vi "Average_P_step.vi"(6 "Averaged P(B) in":dbl[][](array[numeric]), 7 "B array":dbl[](array[numeric]), 9 "Up/Down":bool, 10 "Counter":i8, 11 "Stepped P(B)":dbl[][](array[numeric])) -> (3 "Averaged P(B) out":dbl[][](array[numeric]))   [LabVIEW 2015]
panel:
  out "element":dbl
  out "Offset array dn":dbl[](array[numeric])
  out "P(B) Stepped 2":cluster{"B array":dbl[], "Stepped P(B)":dbl[]}[](graph)
  out "P(B) Averaged":cluster{"B array":dbl[], dbl[]}[](graph)
  out "P(B) Offset removed":cluster{"B array":dbl[], "Stepped P(B)":dbl[]}[](graph)
  out "P(B) Stepped":cluster{"B array":dbl[], dbl[]}[](graph)
  out "OffsetRemoved":dbl[][](array[numeric])
  out "Offset array":dbl[](array[numeric])
  out "size(s)":i32
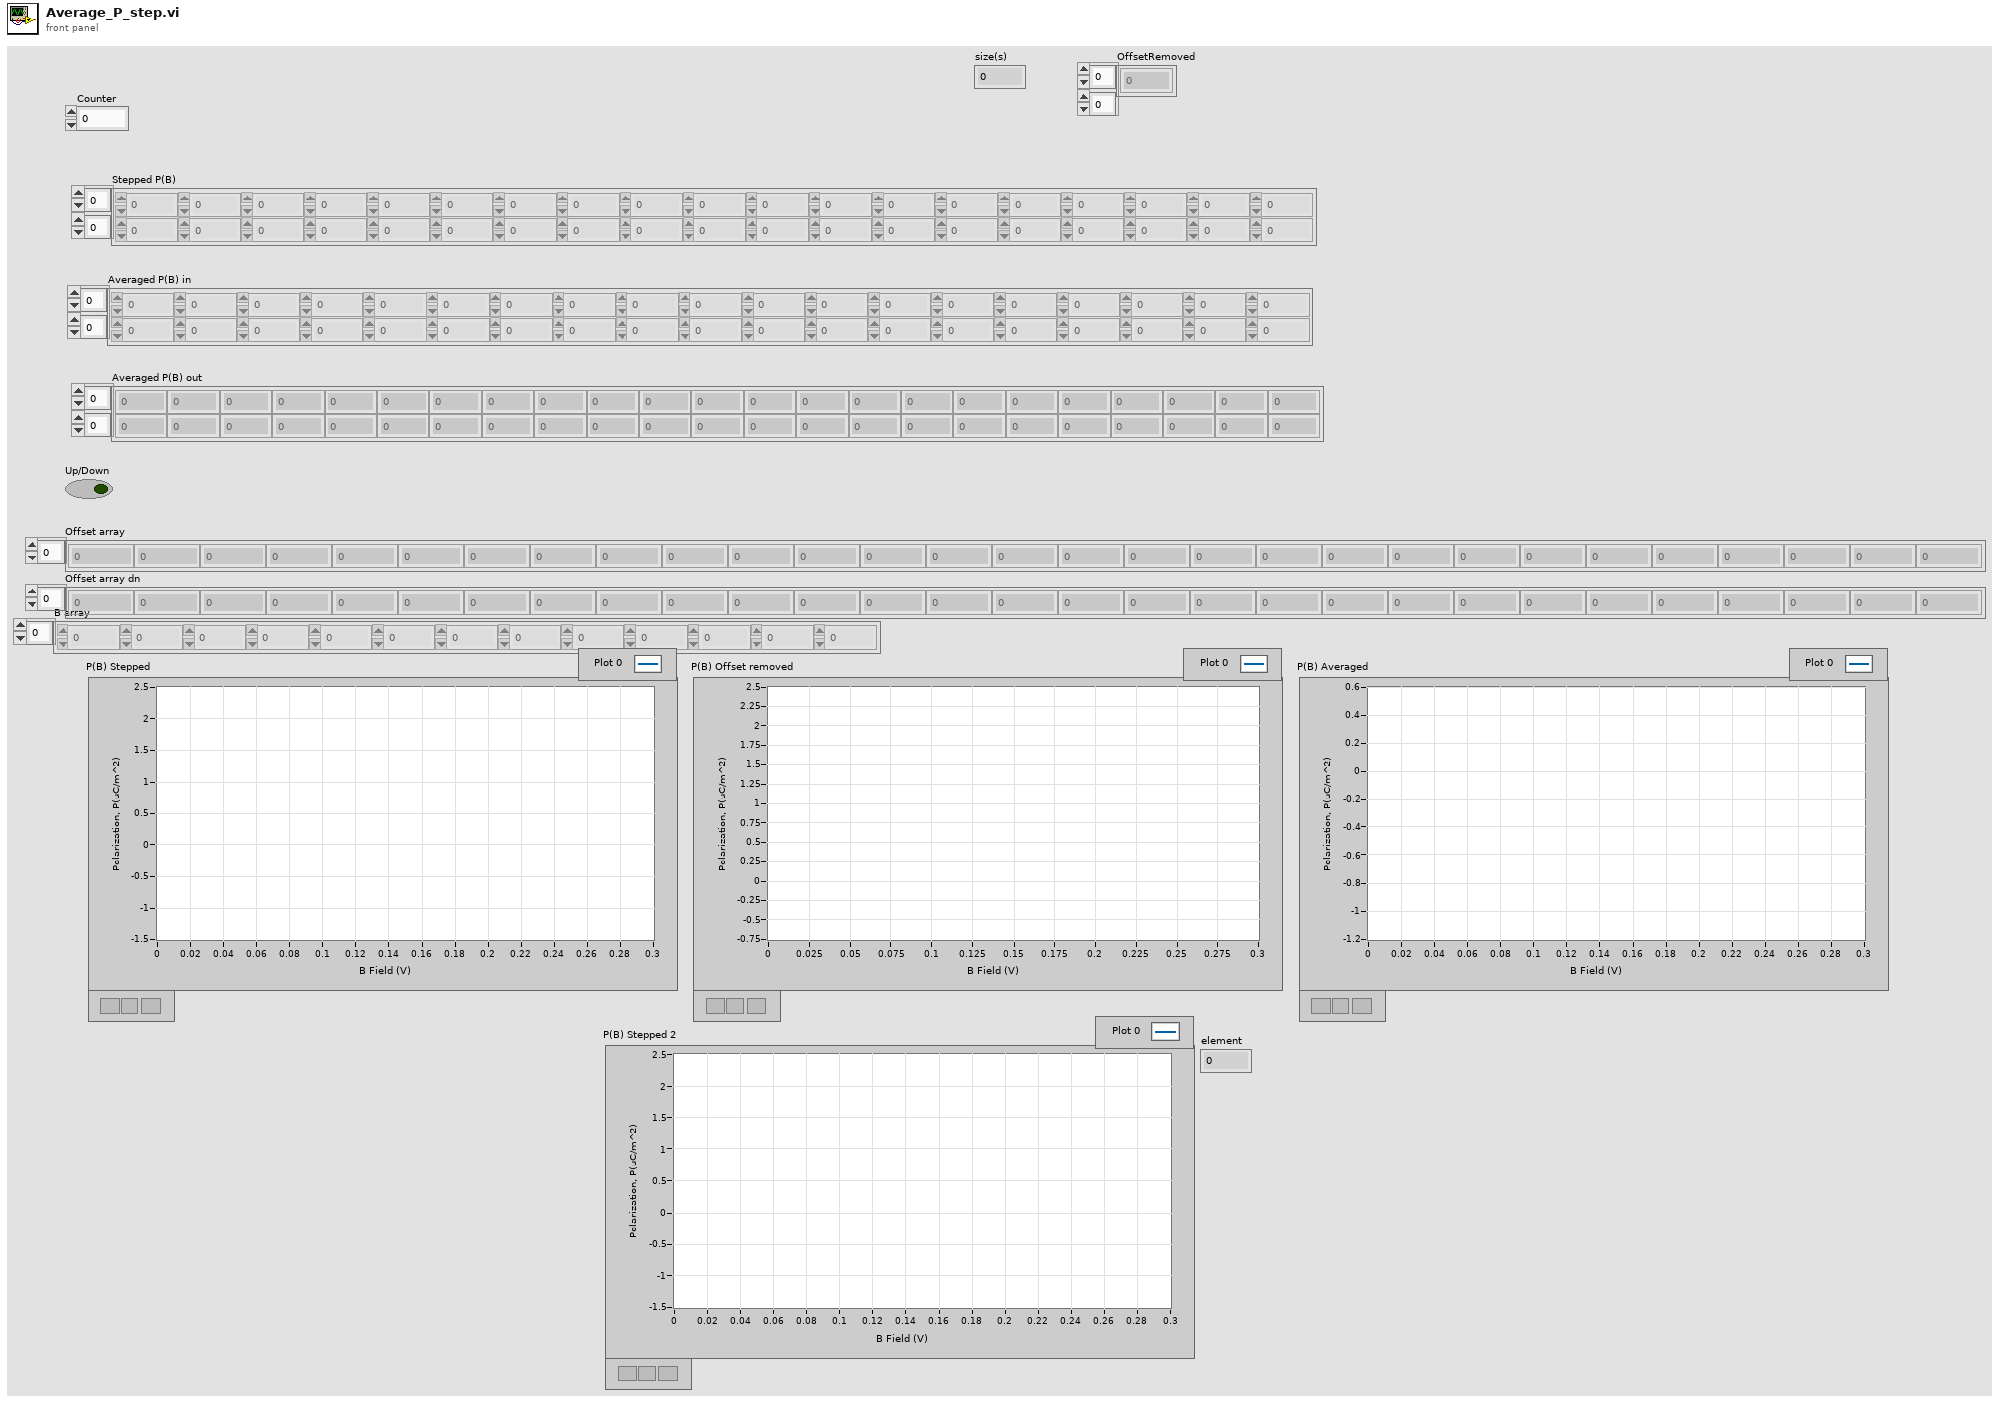
[diagram p1: front panel]
types:
  T1 = cluster{"B array":dbl[], "Averaged P(B) in":dbl[]}
  T2 = cluster{"B array":dbl[], "Averaged P(B) in":dbl[]}[]
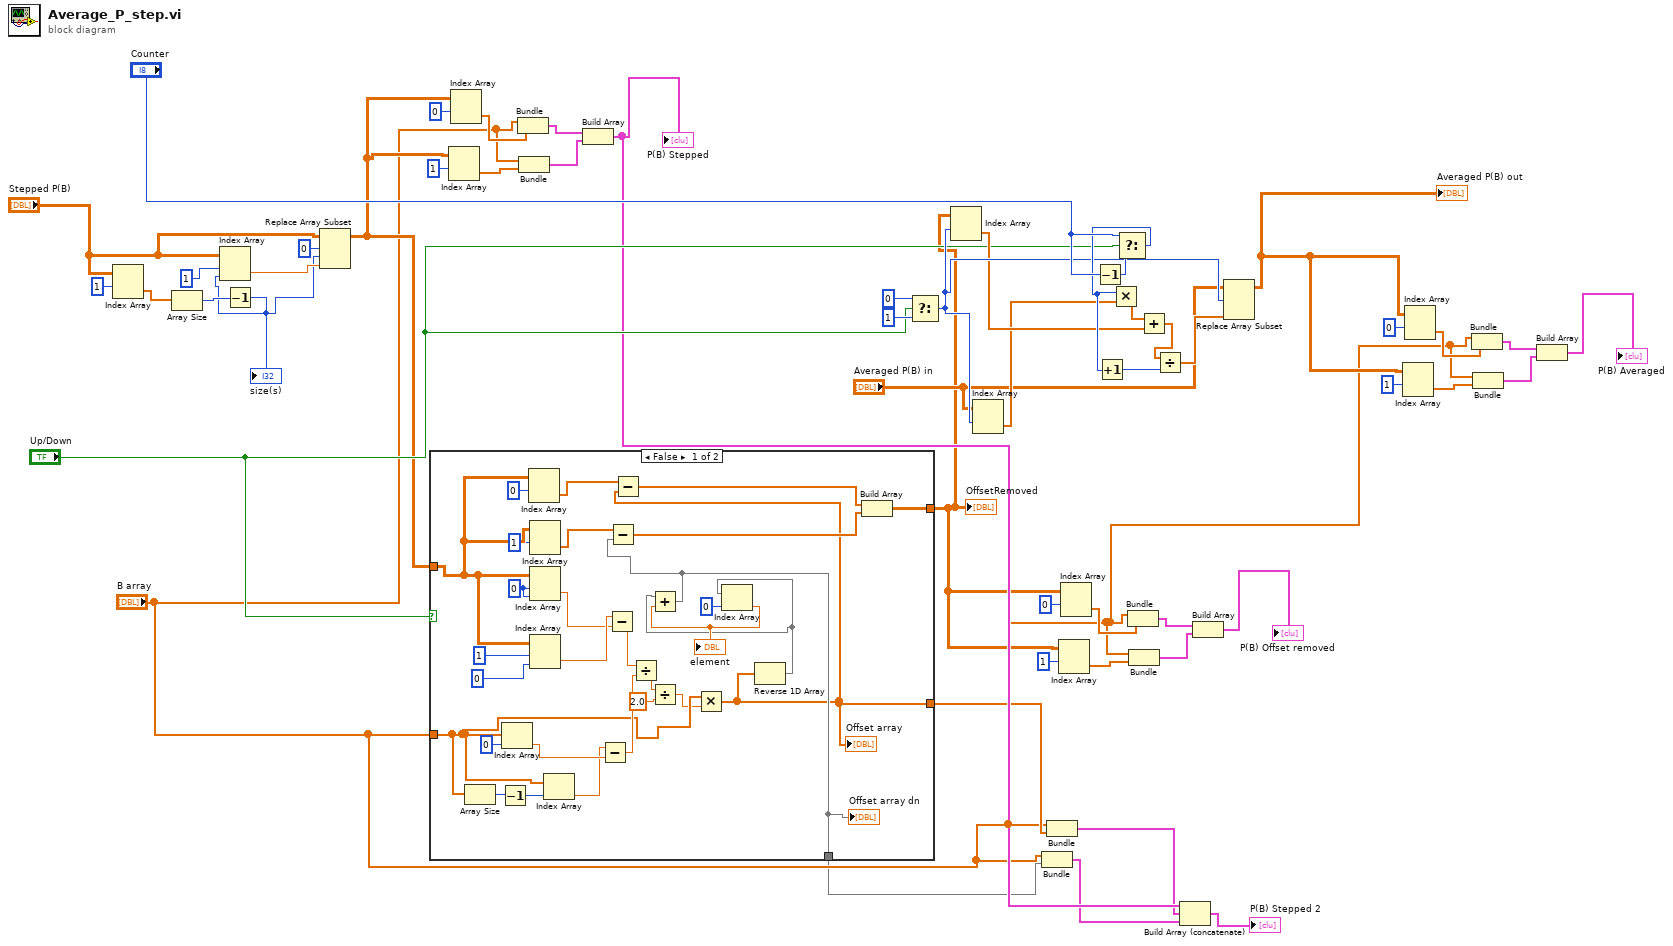
[diagram p0: block diagram]
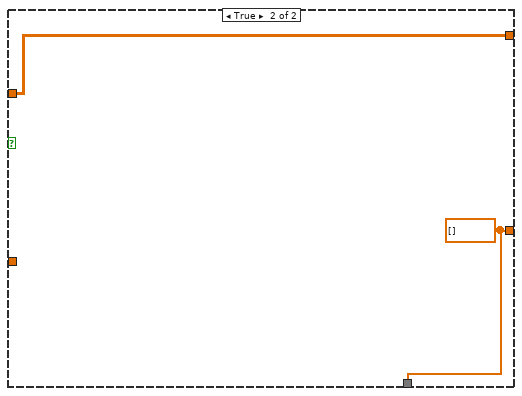
[diagram p2: hidden frame]
diagram:
  n1 = Index Array(array="Stepped P(B)", index (row)=1) -> (element=w39:dbl[])  [unwired: 1 in]
  n2 = Array Size(array=w39) -> (size(s)=w36:i32)
  n3 = Decrement(x=w36) -> (x-1=w33:i32)
  "size(s)" <- w33
  n4 = Index Array(array="Stepped P(B)", index (row)=1, index (col)=w33) -> (element=w37:dbl)
  n5 = Replace Array Subset(array="Stepped P(B)", new element=w37, index (row)=0, index (col)=w33) -> (w9:dbl[][])
  n6 = case shown="False" "Up/Down" {
    tunnel: w9 -> [w73 w83]
    tunnel: "B array" -> [w60 _]
    tunnel: [w61 w83] -> w1
    tunnel: [w54 w82] -> w7
    tunnel: [w55 w82] -> w5
    frame False {
      w81 = 0 ("index (row)")
      n7 = Array Size(array=w60) -> (size(s)=w66:i32)
      n8 = Decrement(x=w66) -> (x-1=w75:i32)
      n9 = Index Array(array=w60, index=0) -> (element=w74:dbl)
      n10 = Index Array(array=w73, index (row)=0) -> (element=w65:dbl[])  [unwired: 1 in]
      n11 = Index Array(array=w73, index (row)=1) -> (element=w64:dbl[])  [unwired: 1 in]
      n12 = Index Array(array=w73, index (row)=w81, index (col)=w81) -> (element=w77:dbl)
      n13 = Index Array(array=w73, index (row)=1, index (col)=0 ("index (row)")) -> (element=w78:dbl)
      n14 = Index Array(array=w60, index=w75) -> (element=w58:dbl)
      n15 = Subtract(x=w58, y=w74) -> (x-y=w69:dbl)
      n16 = Subtract(x=w78, y=w77) -> (x-y=w70:dbl)
      n17 = Divide(x=w70, y=w69) -> (x/y=w68:dbl)
      n18 = Divide(x=w68, y=2.0) -> (x/y=w59:dbl)
      n19 = Multiply(x=w60, y=w59) -> (x*y=w54:dbl[])
      "Offset array" <- w54
      n20 = Subtract(x=w65, y=w54) -> (x-y=w63:dbl[])
      n21 = Reverse 1D Array(array=w54) -> (reversed array=w53:dbl[])
      n22 = Index Array(array=w53, index=0) -> (element=w56:dbl)
      "element" <- w56
      n23 = Add(x=w53, y=w56) -> (x+y=w55:dbl[])
      "Offset array dn" <- w55
      n24 = Subtract(x=w64, y=w55) -> (x-y=w62:dbl[])
      n25 = Build Array(w63, w62) -> (w61:dbl[][])
    }
    frame True {
      w82 = dbl[] []
    }
  }
  "OffsetRemoved" <- w1
  n26 = Index Array(array=w9, index (row)=1) -> (element=w27:dbl[])  [unwired: 1 in]
  n27 = Index Array(array=w9, index (row)=0) -> (element=w28:dbl[])  [unwired: 1 in]
  n28 = Bundle("B array"="B array", "Stepped P(B)"=w28) -> (w26:cluster{"B array":dbl[], "Stepped P(B)":dbl[]})  [unwired: 1 in]
  n29 = Bundle("B array"="B array", "Stepped P(B)"=w27) -> (w25:cluster{"B array":dbl[], "Stepped P(B)":dbl[]})  [unwired: 1 in]
  n30 = Build Array(w26, w25) -> (w8:cluster{"B array":dbl[], "Stepped P(B)":dbl[]}[])
  "P(B) Stepped" <- w8
  n31 = Select(t=0, s="Up/Down", f=1) -> (s? t:f=w48:i32)
  n32 = Index Array(array=w1, index (row)=w48) -> (element=w47:dbl[])  [unwired: 1 in]
  n33 = Index Array(array="Averaged P(B) in", index (row)=w48) -> (element=w46:dbl[])  [unwired: 1 in]
  n34 = Bundle("B array"="B array", w5) -> (w3:cluster{"B array":dbl[], dbl[]})  [unwired: 1 in]
  n35 = Bundle("B array"="B array", w7) -> (w4:cluster{"B array":dbl[], dbl[]})  [unwired: 1 in]
  n36 = Index Array(array=w1, index (row)=1) -> (element=w21:dbl[])  [unwired: 1 in]
  n37 = Index Array(array=w1, index (row)=0) -> (element=w20:dbl[])  [unwired: 1 in]
  n38 = Decrement(x="Counter") -> (x-1=w50:i8)
  n39 = Select(t="Counter", s="Up/Down", f=w50) -> (s? t:f=w51:i8)
  n40 = Increment(x=w51) -> (x+1=w42:i8)
  n41 = Multiply(x=w51, y=w46) -> (x*y=w41:dbl[])
  n42 = Bundle("B array"="B array", "Stepped P(B)"=w20) -> (w22:cluster{"B array":dbl[], "Stepped P(B)":dbl[]})  [unwired: 1 in]
  n43 = Bundle("B array"="B array", "Stepped P(B)"=w21) -> (w23:cluster{"B array":dbl[], "Stepped P(B)":dbl[]})  [unwired: 1 in]
  n44 = Add(x=w41, y=w47) -> (x+y=w43:dbl[])
  n45 = Divide(x=w43, y=w42) -> (x/y=w49:dbl[])
  n46 = Build Array (concatenate)(w8, w4, w3) -> (→"P(B) Stepped 2":cluster{"B array":dbl[], "Stepped P(B)":dbl[]}[])
  n47 = Build Array(w22, w23) -> (→"P(B) Offset removed":cluster{"B array":dbl[], "Stepped P(B)":dbl[]}[])
  n48 = Replace Array Subset(array="Averaged P(B) in", new element=w49, index (row)=w48) -> (w10:dbl[][])  [unwired: 1 in]
  "Averaged P(B) out" <- w10
  n49 = Index Array(array=w10, index (row)=1) -> (element=w14:dbl[])  [unwired: 1 in]
  n50 = Index Array(array=w10, index (row)=0) -> (element=w15:dbl[])  [unwired: 1 in]
  n51 = Bundle("B array"="B array", "Averaged P(B) in"=w15) -> (w13:T1)  [unwired: 1 in]
  n52 = Bundle("B array"="B array", "Averaged P(B) in"=w14) -> (w12:T1)  [unwired: 1 in]
  n53 = Build Array(w13, w12) -> (→"P(B) Averaged":T2)
